vi "Start Testing.vi"(8 "error in (no error)":errorcluster, 10 "Test Settings":T1 {"Lateral Load Cell Sensitivity" format="%.6f"; "Axial Load Cell Sensitivity" format="%.6f"}, 11 "Context in":refnum<class "Context.lvclass">) -> (0 "error out":errorcluster, 3 "Context out":refnum<class "Context.lvclass">)   [LabVIEW 2015, in "Context.lvclass"]
uses:
  Context.lvclass
  Typedefs/TestSettings.ctl
  Common_RT_FAILC/DataTypes/FATypes.ctl
  Context.lvclass/Context.ctl
  States/State/State.lvclass
  Model/Model/Model.lvclass
  Typedefs/FAMT Typedefs.lvlib
  Common_RT_FAILC/RTFAILC.lvlib
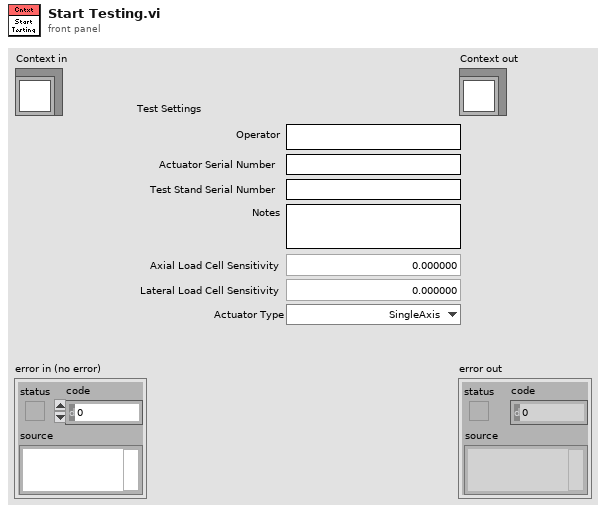
[diagram p1: front panel]
types:
  T1 = typedef "FAMT Typedefs.lvlib/TestSettings.ctl" = cluster{"Operator":string, "Notes":string, "Actuator Serial Number":string, "Test Stand Serial Number":string, "Axial Load Cell Sensitivity":dbl, "Lateral Load Cell Sensitivity":dbl, "Actuator Type":T2}
  T2 = typedef "RTFAILC.lvlib/FATypes.ctl" = enum16{"SingleAxis", "LateralDualAxis", "CrossLateralDualAxis"}
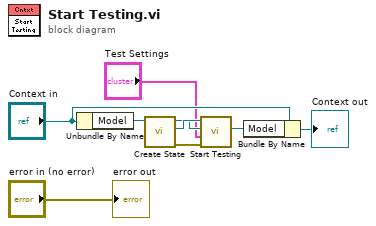
[diagram p0: block diagram]
diagram:
  n1 = Unbundle By Name("Context in") -> ("Model"=w8:refnum<class "Model.lvclass">)
  n2 = call "Create State.vi"("Model in"=w8) -> ("error out"=w2:errorcluster, "State"=w4:refnum<class "State.lvclass">, "Model out"=w3:refnum<class "Model.lvclass">)  [unwired: 8 in]
  n3 = call-dynamic "Start Testing.vi"("error in (no error)"=w2, "Scan Settings"="Test Settings", "Model in"=w3, "State in"=w4) -> ("Model out"=w5:refnum<class "Model.lvclass">)  [unwired: 5 in, 2 out]
  n4 = Bundle By Name(cluster="Context in", "Model"=w5) -> (→"Context out":refnum<class "Context.lvclass">)
  "error out" <- "error in (no error)"
